vi "Savitzky-Golay Filter (DBL).vi"(8 "Weight":dbl[](array[numeric]), 9 "polynomial order":i32=3, 10 "side points":i32=6, 11 "X":dbl[](array[numeric])) -> (0 "error":i32, 3 "Filtered X":dbl[](array[numeric]))   [LabVIEW 2010, in "NI_AALBase.lvlib"]
doc: "Filters the input data sequence<B> X</B> using a Savitzky-Golay FIR smoothing filter. Wire data to the <B>X</B> input to determine the polymorphic instance to use or manually select the instance."
uses:
  NI_AALBase.lvlib
  lvanlys.dll
panel:
  # "Savitzky-Golay Filter"
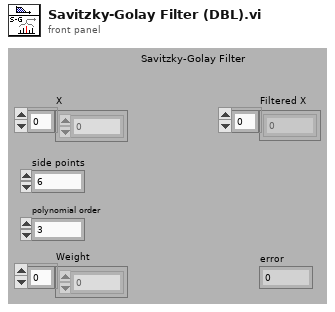
[diagram p1: front panel]
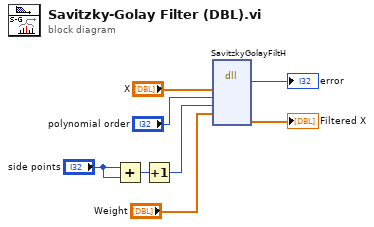
[diagram p0: block diagram]
diagram:
  n1 = Add(x="side points", y="side points") -> (x+y=w3:i32)
  n2 = Increment(x=w3) -> (x+1=w1:i32)
  n3 = dll-call lib="C:/Program Files/National Instruments/LabVIEW 2010/resource/lvanlys.*" fn="SavitzkyGolayFiltH"("xH"="X", "polyOrder"="polynomial order", "frameSize"=w1, "weight"="Weight") -> (→"error":i32, "yH"=→"Filtered X":dbl[])  [unwired: 8 in, 2 out]
